vi "Check_Traverse_move_PN.vi"(0 "Current position":sgl[](array[numeric])=[0.0, 0.0, 0.0] format="%.2f", 1 "Traverse Name":string, 2 "Full Check":bool, 5 "New Position":sgl[](array[numeric])=[0.0, 0.0, 0.0] format="%.2f", 7 "Model       Roll      Pitch       Yaw (deg)":sgl[](array[numeric]) format="%#.2f") -> (6 "Position At Crash":sgl[](array[numeric]) format="%.2f", 10 "Steps":sgl[][](array[numeric]) format="%.2f", 15 "Error Comments":string)   [LabVIEW 2016]
uses:
  Collision_Detection/Triangles/EnFlo specific/Collision Mode.ctl
panel:
  # "X                Y                   Z"
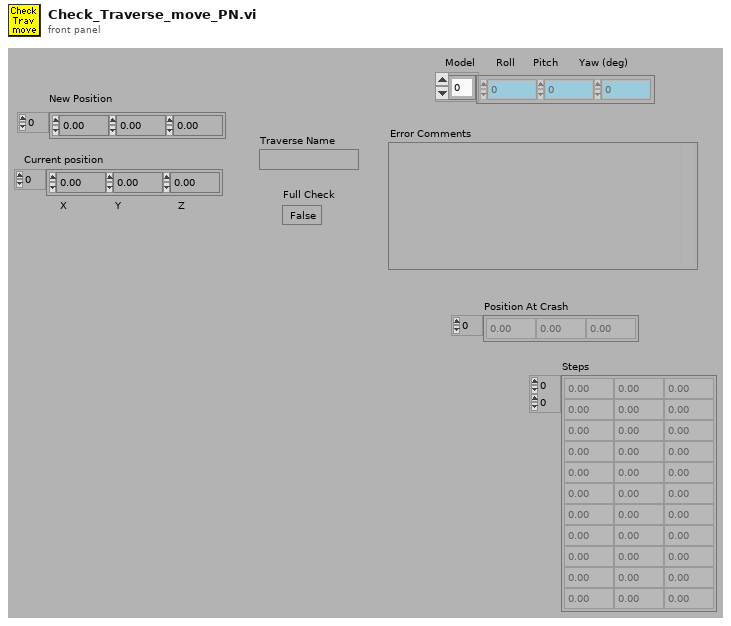
[diagram p1: front panel]
types:
  T1 = enum16{"To Traverse Coordinates", "To User Coordinates"}
  T2 = typedef "Collision Mode.ctl" = enum16{"Traverse - Tunnel", "Traverse - Model", "Traverse - Fixed objects", "Traverse - Traverse", "Traverse - All"}
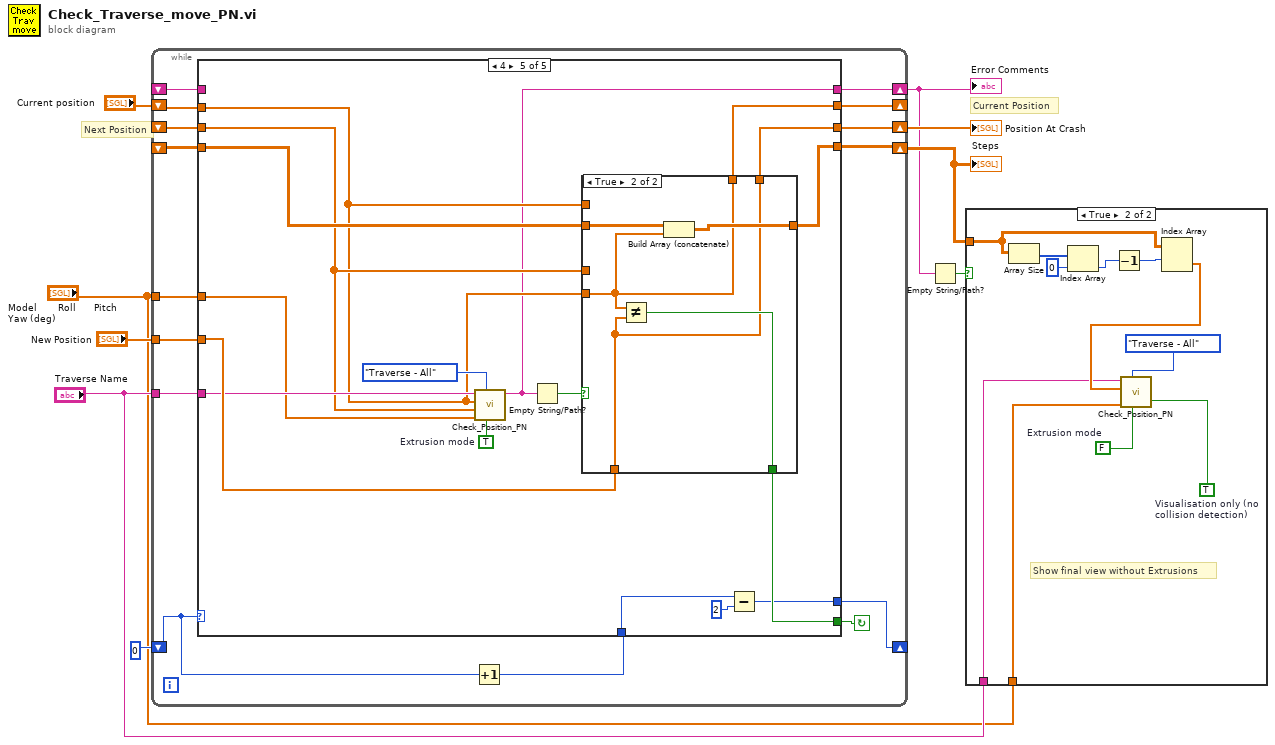
[diagram p0: block diagram]
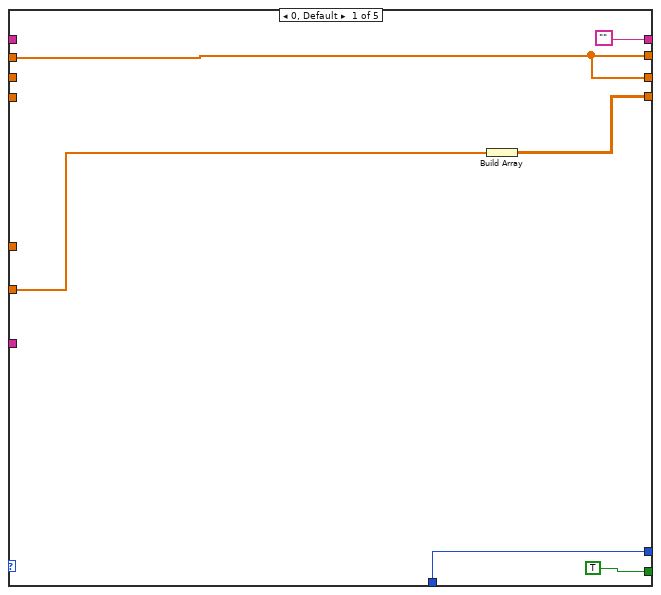
[diagram p3: hidden frame]
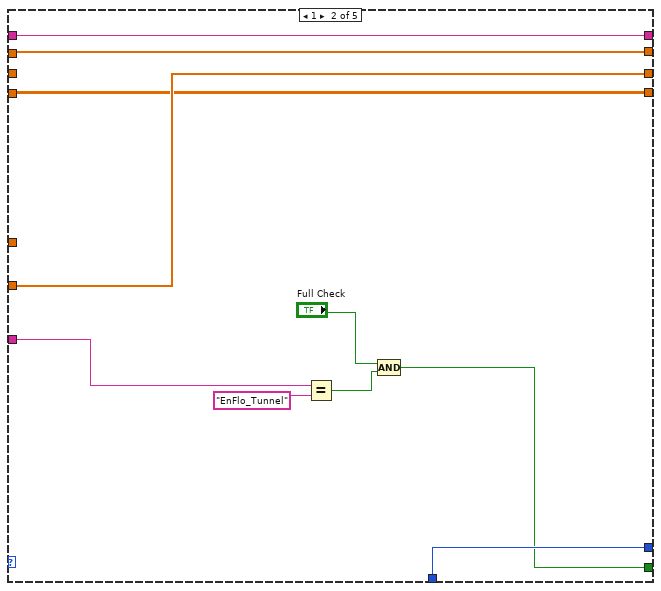
[diagram p4: hidden frame]
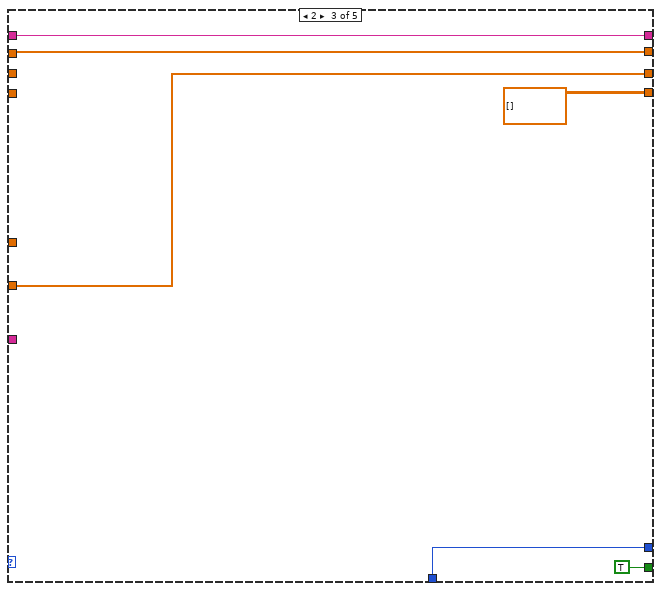
[diagram p5: hidden frame]
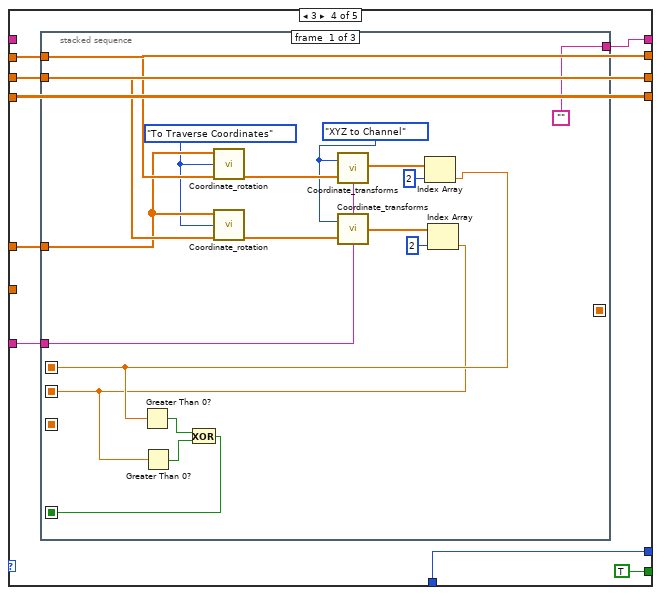
[diagram p6: hidden frame]
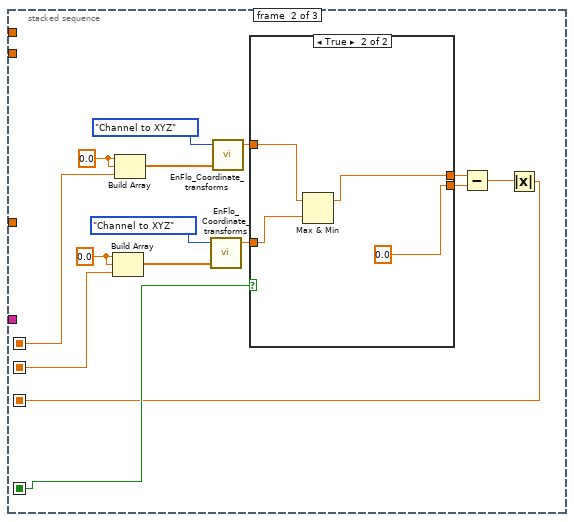
[diagram p7: hidden frame]
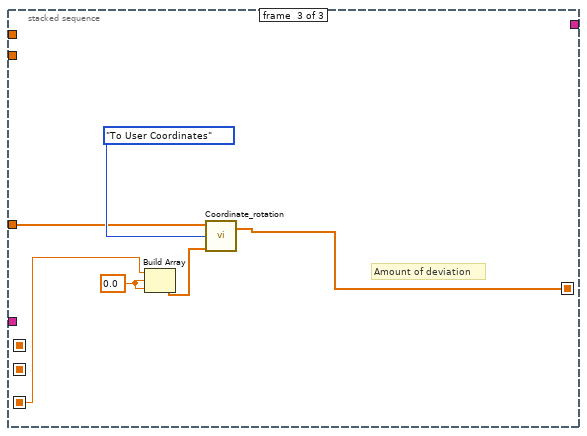
[diagram p9: hidden frame]
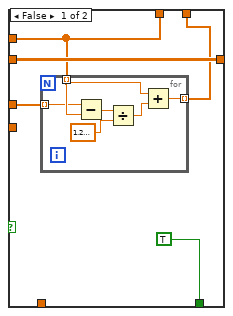
[diagram p10: hidden frame]
diagram:
  # "Current Position"
  # "Next Position"
  n1 = while {
    shift-left: _ -> [w11]
    shift-right: [w10] -> w5
    tunnel: "Model       Roll      Pitch       Yaw (deg)" -> [w12]
    tunnel: "New Position" -> [w13]
    shift-left: _ -> [w15]
    shift-right: [w16] -> w4
    shift-left: 0 -> [w19]
    shift-right: [w18] -> _
    tunnel: "Traverse Name" -> [w20]
    shift-left: _ -> [w14]
    shift-right: [w22] -> w6
    shift-left: "Current position" -> [w24]
    shift-right: [w23] -> _
    stop <- w21 continue-if-true
    n2 = Increment(x=w19) -> (x+1=w17:i32)
    n3 = case shown="4" w19 {
      tunnel: w24 -> [w25 w39 w45 w52 w101]
      tunnel: [w25 w39 w45 w52 w111] -> w23
      tunnel: [w25 w33 w43 w51 w110] -> w22
      tunnel: [TRUE ("Box Inside") w35 TRUE ("Box Inside") TRUE ("Box Inside") w112] -> w21
      tunnel: w20 -> [_ w36 _ w49 w104]
      tunnel: [w27 w38 w44 w48 w108] -> w18
      tunnel: w17 -> [w27 w38 w44 w48 w107]
      tunnel: ["" w40 w46 w54 w100] -> w16
      tunnel: w15 -> [_ w40 w46 _ _]
      tunnel: w14 -> [_ _ _ w51 w103]
      tunnel: w13 -> [w30 w33 w43 _ w113]
      tunnel: w12 -> [_ _ _ w50 w102]
      tunnel: w11 -> [_ w32 _ w47 w116]
      tunnel: [w29 w32 sgl[][] [] w47 w115] -> w10
      frame 0, Default {
        n4 = Build Array(w30) -> (w29:sgl[][])
      }
      frame 1 {
        n5 = Equal?(x=w36, y="EnFlo_Tunnel") -> (x = y?=w31:bool)
        n6 = Compound Arithmetic op=AND("Full Check", w31) -> (w35:bool)
      }
      frame 2 {
      }
      frame 3 {
        n7 = stacked-sequence {
          seq-local: [w57 _ _] -> [_ w87 _]
          seq-local: [w56 _ _] -> [_ w86 _]
          seq-local: [w55 _ _] -> [_ w77 _]
          seq-local: [_ w73 _] -> [_ _ w96]
          seq-local: [_ _ w94] -> [_ _ _]
          tunnel: ["" _ _] -> w54
          tunnel: w52 -> [w70 _ _]
          tunnel: w51 -> [w68 _ _]
          tunnel: w50 -> [w67 _ w95]
          tunnel: w49 -> [w66 _ _]
          frame #0 {
            w64 = enum16{"XYZ to Channel", "Channel to XYZ"}."XYZ to Channel" ("Mode")
            w65 = T1."To Traverse Coordinates" ("Mode")
            n8 = call "Coordinate_rotation.vi"("Roll-Pitch-Yaw"=w67, "Input Position"=w70, "Mode"=w65) -> ("Output Position"=w71:sgl[])  [unwired: 2 in, 1 out]
            n9 = call "Coordinate_rotation.vi"("Roll-Pitch-Yaw"=w67, "Input Position"=w68, "Mode"=w65) -> ("Output Position"=w69:sgl[])  [unwired: 2 in, 1 out]
            n10 = call "Coordinate_transforms.vi"("Traverse Name"=w66, "Input"=w71, "Mode"=w64) -> ("Output"=w63:sgl[])
            n11 = call "Coordinate_transforms.vi"("Traverse Name"=w66, "Input"=w69, "Mode"=w64) -> ("Output"=w60:sgl[])
            n12 = Index Array(array=w63, index=2) -> (element=w57:sgl)
            n13 = Greater Than 0?(x=w57) -> (x > 0?=w59:bool)
            n14 = Index Array(array=w60, index=2) -> (element=w56:sgl)
            n15 = Greater Than 0?(x=w56) -> (x > 0?=w58:bool)
            n16 = Exclusive Or(1:w58, 2:w59) -> (0:w55:bool)
          }
          frame #1 {
            w80 = 0.0 ("element")
            w85 = 0.0 ("element")
            n17 = Build Array(w80, w80, w86) -> (w82:dbl[])
            n18 = Build Array(w85, w85, w87) -> (w83:dbl[])
            n19 = call "EnFlo_Coordinate_transforms.vi"("Input"=w82, "Mode"=enum16{"XYZ to Channel", "Channel to XYZ"}."Channel to XYZ") -> ("X theta"=w78:dbl)  [unwired: 3 out]
            n20 = call "EnFlo_Coordinate_transforms.vi"("Input"=w83, "Mode"=enum16{"XYZ to Channel", "Channel to XYZ"}."Channel to XYZ") -> ("X theta"=w79:dbl)  [unwired: 3 out]
            n21 = case shown="True" w77 {
              tunnel: w79 -> [w89 w92]
              tunnel: w78 -> [w88 w93]
              tunnel: [w88 0.0 ("element")] -> w76
              tunnel: [w89 w91] -> w75
              frame False {
              }
              frame True {
                n22 = Max & Min(x=w92, y=w93) -> (max(x,y)=w91:dbl)  [unwired: 1 out]
              }
            }
            n23 = Subtract(x=w75, y=w76) -> (x-y=w74:dbl)
            n24 = Absolute Value(x=w74) -> (abs(x)=w73:dbl)
          }
          frame #2 {
            w98 = 0.0 ("Input Element")
            # "Amount of deviation"
            n25 = Build Array(w96, w98, w98) -> (w97:dbl[])
            n26 = call "Coordinate_rotation.vi"("Roll-Pitch-Yaw"=w95, "Input Position"=w97, "Mode"=T1."To User Coordinates") -> ("Output Position"=w94:sgl[])  [unwired: 2 in, 1 out]
          }
        }
      }
      frame 4 {
        w105 = TRUE  # Extrusion mode
        n27 = call "Check_Position_PN.vi"("Extrusion mode"=w105, "Collision mode"=Collision_Mode."Traverse - All", "Model Rotation (deg)"=w102, "Traverse extruded position"=w103, "Position to check"=w101, "Traverse Name"=w104) -> ("Error Comments"=w100:string)  [unwired: 2 in, 2 out]
        n28 = Empty String/Path?(string/path=w100) -> (empty?=w114:bool)
        n29 = case shown="True" w114 {
          tunnel: w116 -> [w121 w132]
          tunnel: w101 -> [_ w129]
          tunnel: [w121 w131] -> w115
          tunnel: w113 -> [_ w128]
          tunnel: [TRUE w130] -> w112
          tunnel: [w119 w129] -> w111
          tunnel: [w117 w128] -> w110
          tunnel: w101 -> [w119 _]
          tunnel: w103 -> [w118 _]
          frame False {
            n30 = for {
              tunnel: w119 -> [w123] mode=indexing
              tunnel: w118 -> [w122] mode=indexing
              tunnel: [w124] -> w117 mode=indexing
              n31 = Subtract(x=w122, y=w123) -> (x-y=w127:sgl)
              n32 = Divide(x=w127, y=sgl 1.2) -> (x/y=w125:sgl)
              n33 = Add(x=w123, y=w125) -> (x+y=w124:sgl)
            }
          }
          frame True {
            n34 = Not Equal?(x=w129, y=w128) -> (x != y?=w130:bool)
            n35 = Build Array (concatenate)(w132, w129) -> (w131:sgl[][])
          }
        }
        n36 = Subtract(x=w107, y=2) -> (x-y=w108:i32)
      }
    }
  }
  "Error Comments" <- w4
  "Position At Crash" <- w6
  "Steps" <- w5
  n37 = Empty String/Path?(string/path=w4) -> (empty?=w3:bool)
  n38 = case shown="True" w3 {
    tunnel: w5 -> [_ w139]
    tunnel: "Model       Roll      Pitch       Yaw (deg)" -> [_ w136]
    tunnel: "Traverse Name" -> [_ w137]
    frame False {
    }
    frame True {
      w134 = FALSE  # Extrusion mode
      w135 = TRUE  # Visualisation only (no collision detection)
      # "Show final view without Extrusions"
      n39 = Array Size(array=w139) -> (size(s)=w143:i32[])
      n40 = Index Array(array=w143, index=0) -> (element=w141:i32)
      n41 = Decrement(x=w141) -> (x-1=w140:i32)
      n42 = Index Array(array=w139, index (row)=w140) -> (element=w138:sgl[])  [unwired: 1 in]
      n43 = call "Check_Position_PN.vi"("Visualisation only (no collision detection)"=w135, "Extrusion mode"=w134, "Collision mode"=Collision_Mode."Traverse - All", "Model Rotation (deg)"=w136, "Position to check"=w138, "Traverse Name"=w137) -> ()  [unwired: 2 in, 3 out]
    }
  }
